vi "Handle LS Data.vi"(8 "Initial LS Data":T1={"Total Cycles"=[0, 0, 0, 0, 0, 0], "Steps"=[0, 0, 0, 0, 0, 0], "Anomalies Total"=[0, 0, 0, 0, 0, 0], "Cycles"=[0, 0, 0, 0, 0, 0], "Anomalies/Cycle"=[0, 0, 0, 0, 0, 0], "Anomalies (Last Cycle)"=[0, 0, 0, 0, 0, 0], "Opens"=[0, 0, 0, 0, 0, 0]} {"Opens" format="%#.0f"; "Anomalies (Last Cycle)" format="%#.0f"; "Anomalies/Cycle" format="%#.0f"; "Cycles" format="%#.0f"; "Anomalies Total" format="%#.0f"; "Steps" format="%#.0f"; "Total Cycles" format="%#.0f"}, 11 "FPGA LS Data":T1={"Total Cycles"=[0, 0, 0, 0, 0, 0], "Steps"=[0, 0, 0, 0, 0, 0], "Anomalies Total"=[0, 0, 0, 0, 0, 0], "Cycles"=[0, 0, 0, 0, 0, 0], "Anomalies/Cycle"=[0, 0, 0, 0, 0, 0], "Anomalies (Last Cycle)"=[0, 0, 0, 0, 0, 0], "Opens"=[0, 0, 0, 0, 0, 0]} {"Opens" format="%#.0f"; "Anomalies (Last Cycle)" format="%#.0f"; "Anomalies/Cycle" format="%#.0f"; "Cycles" format="%#.0f"; "Anomalies Total" format="%#.0f"; "Steps" format="%#.0f"; "Total Cycles" format="%#.0f"}) -> (3 "LS Data":T1 {"Opens" format="%#.0f"; "Anomalies (Last Cycle)" format="%#.0f"; "Anomalies/Cycle" format="%#.0f"; "Cycles" format="%#.0f"; "Anomalies Total" format="%#.0f"; "Steps" format="%#.0f"; "Total Cycles" format="%#.0f"})   [LabVIEW 2019]
uses:
  Type Defs/LS Data.ctl
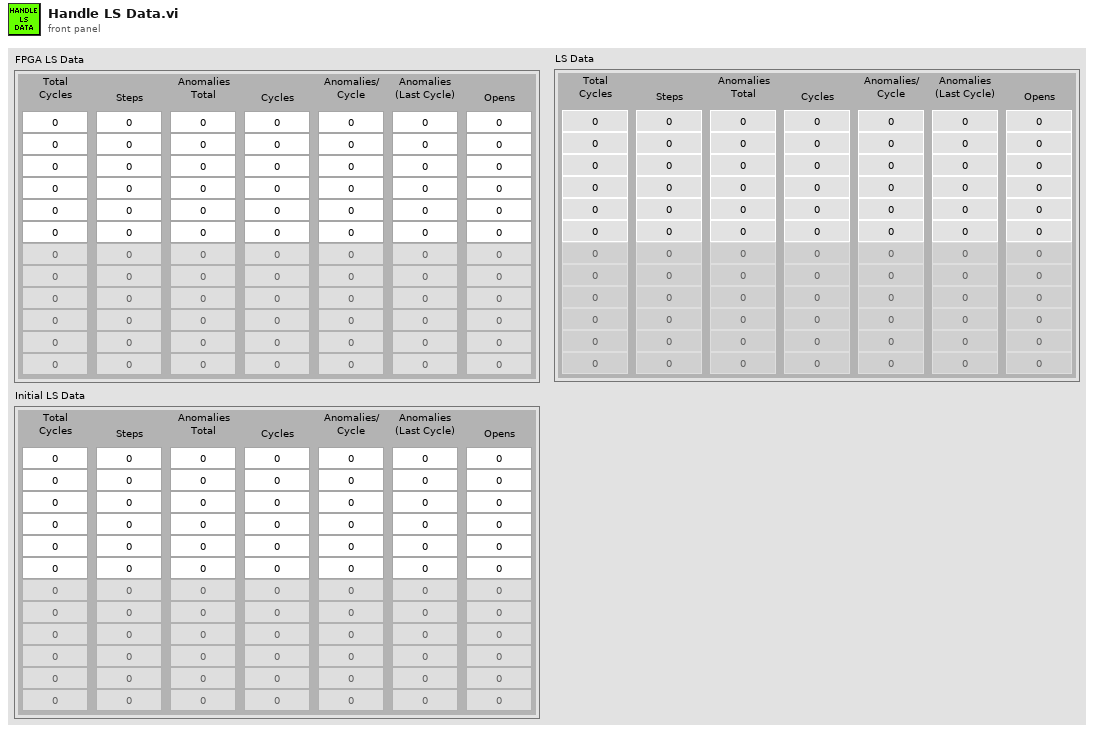
[diagram p1: front panel]
types:
  T1 = typedef "LS Data.ctl" = cluster{"Total Cycles":u32[], "Steps":u32[], "Anomalies Total":i32[], "Cycles":u32[], "Anomalies/Cycle":i32[], "Anomalies (Last Cycle)":i32[], "Opens":i32[]}
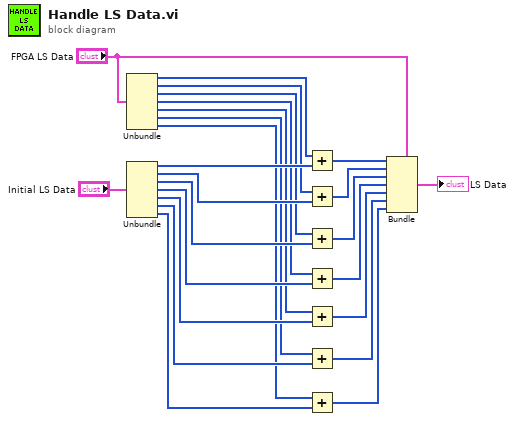
[diagram p0: block diagram]
diagram:
  n1 = Unbundle("FPGA LS Data") -> ("Total Cycles"=w7:u32[], "Steps"=w6:u32[], "Anomalies Total"=w5:i32[], "Cycles"=w4:u32[], "Anomalies/Cycle"=w3:i32[], "Anomalies (Last Cycle)"=w2:i32[], "Opens"=w1:i32[])
  n2 = Unbundle("Initial LS Data") -> ("Total Cycles"=w14:u32[], "Steps"=w15:u32[], "Anomalies Total"=w16:i32[], "Cycles"=w17:u32[], "Anomalies/Cycle"=w18:i32[], "Anomalies (Last Cycle)"=w19:i32[], "Opens"=w21:i32[])
  n3 = Add(x=w7, y=w14) -> (x+y=w8:u32[])
  n4 = Add(x=w6, y=w15) -> (x+y=w9:u32[])
  n5 = Add(x=w5, y=w16) -> (x+y=w10:i32[])
  n6 = Add(x=w4, y=w17) -> (x+y=w11:u32[])
  n7 = Add(x=w3, y=w18) -> (x+y=w12:i32[])
  n8 = Add(x=w2, y=w19) -> (x+y=w13:i32[])
  n9 = Add(x=w1, y=w21) -> (x+y=w20:i32[])
  n10 = Bundle(cluster="FPGA LS Data", "Total Cycles"=w8, "Steps"=w9, "Anomalies Total"=w10, "Cycles"=w11, "Anomalies/Cycle"=w12, "Anomalies (Last Cycle)"=w13, "Opens"=w20) -> (→"LS Data":T1)
